vi "Wash Display Console View.vi"(8 "error in (no error)":errorcluster, 11 "View Model":T2) -> (0 "error out":errorcluster)   [LabVIEW 2017]
doc: "The Interface via which the wash controller displays the progress of the car wash.\n[Covers: UI3]"
uses:
  Model/Controls/View Model.ctl
  Model/Controls/Shared Model.ctl
  Model/Controls/Views Action.ctl
  Error Handler/Controls/Error Model.ctl
  Error Handler/Controls/Error Message.ctl
  Error Handler/Controls/Error Type.ctl
  Configuration/Controls/Config Model.ctl
  Configuration/Controls/Config DB Message.ctl
  Configuration/Controls/Config DB Command.ctl
  Configuration/Controls/Config DB Overhead.ctl
  Configuration/Controls/Config DB Record.ctl
  Controller/Controls/Controller Model.ctl
  Vehicle Position Simulation View/Controls/Vehicle - Position.ctl
  Controller/Controls/Controller Overhead.ctl
  Controller/Controls/Controller Wash Step.ctl
  Controls/Wash Display - LEDs.ctl
  Controls/Wash Display - GUI References.ctl
  Timing/Controls/Timer - Action.ctl
panel:
  out "Time Remaining":dbl format="%07.2g"
  out "Vehicle Out":bool caption="Vehicle Out of Position"
  out "Wash Entry":bool
  out "Wash LEDs":T1 caption="Car Wash Indicators"
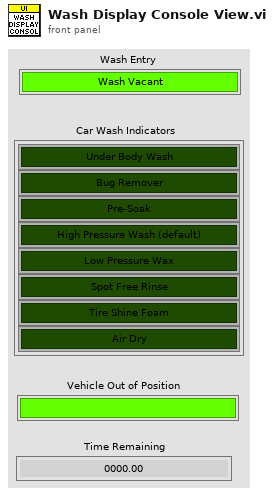
[diagram p1: front panel]
types:
  T1 = typedef "Wash Display - LEDs.ctl" = cluster{"Under Body Wash":bool, "Bug Remover":bool, "Pre-Soak":bool, "High Pressure Wash":bool, "Low Pressure Wax":bool, "Spot Free Rinse":bool, "Tire Shine Foam":bool, "Air Dry":bool}
  T2 = typedef "View Model.ctl" = cluster{"Shared Model":T3, "Error Model":T4, "Config Model":T5, "Controller Model":T6}
  T3 = typedef "Shared Model.ctl" = cluster{"Stop":refnum<user-event>, "Stop DVR":refnum<data-value>, "Views Action":refnum<user-event>}
  T4 = typedef "Error Model.ctl" = cluster{"Error":refnum<user-event>}
  T5 = typedef "Config Model.ctl" = cluster{"Config":refnum<user-event>, "Config DVR":refnum<data-value>}
  T6 = typedef "Controller Model.ctl" = cluster{"Position Change":refnum<user-event>, "Overhead DVR":refnum<data-value>, "Wash Cycle Start":refnum<user-event>, "Wash Step Start":refnum<user-event>, "Out Of Position":refnum<user-event>}
  T7 = typedef "Wash Display - GUI References.ctl" = cluster{"Time Remaining":refnum<vi>, "Vehicle Out":refnum<vi>, "Wash LEDs":refnum<vi>, "Wash Entry":refnum<vi>}
  T8 = typedef "Timer - Action.ctl" = enum16{"Start", "Get Time", "Pause", "UnPause"}
  T9 = typedef "Error Type.ctl" = enum16{"Minor Error", "Wash Cycle Error", "System Error", "Unknown"}
  T10 = typedef "Views Action.ctl" = enum16{"Initial", "Wash Cycle Start", "Wash Cycle Complete", "Wash Exit", "Wash Abort/Terminate", "Wash Step Start", "Wash Step Execute", "Wash Step Complete"}
  T11 = typedef "Controller Wash Step.ctl" = enum16{"None", "Under Body Wash", "Bug Remover", "Pre-Soak", "High Pressure Wash", "Low Pressure Wax", "Spot Free Rinse", "Tire Shine Foam", "Air Dry"}
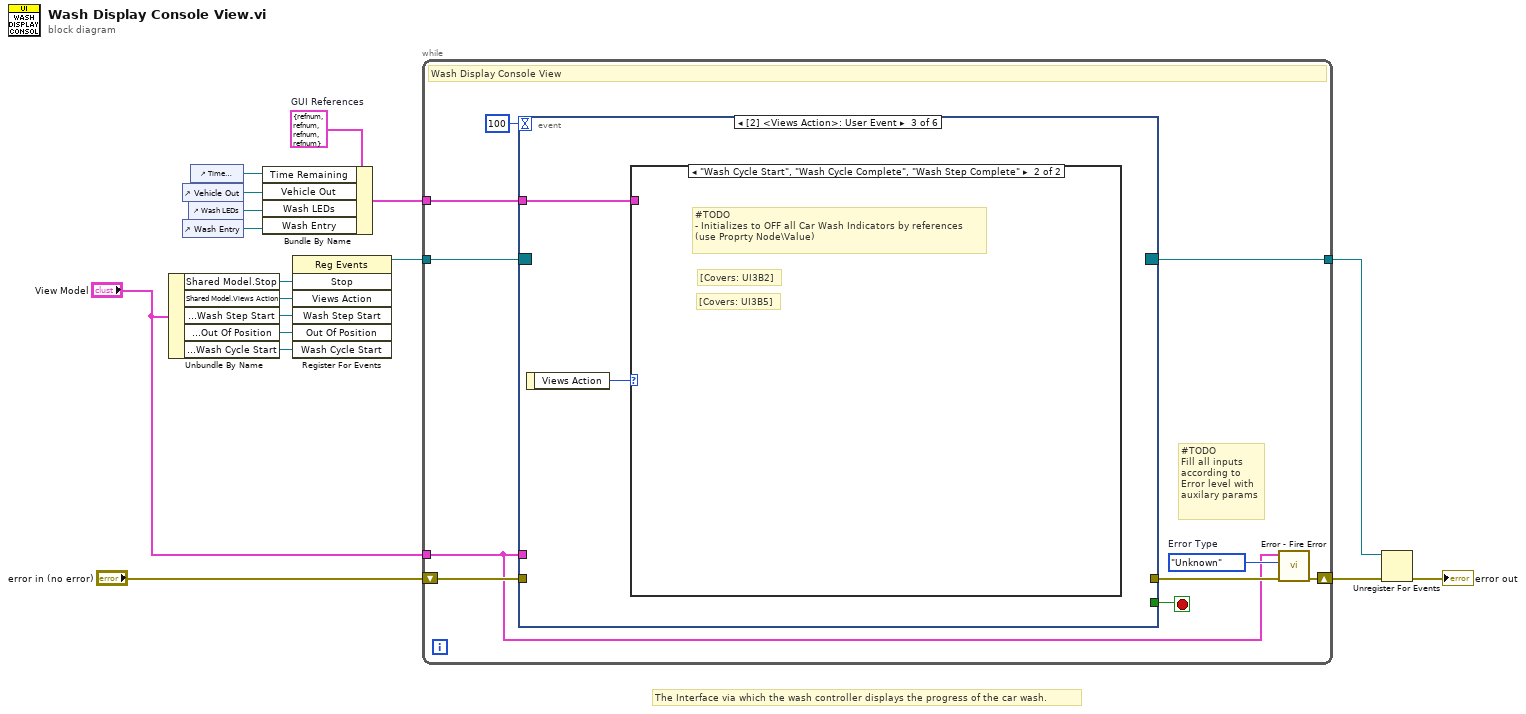
[diagram p0: block diagram]
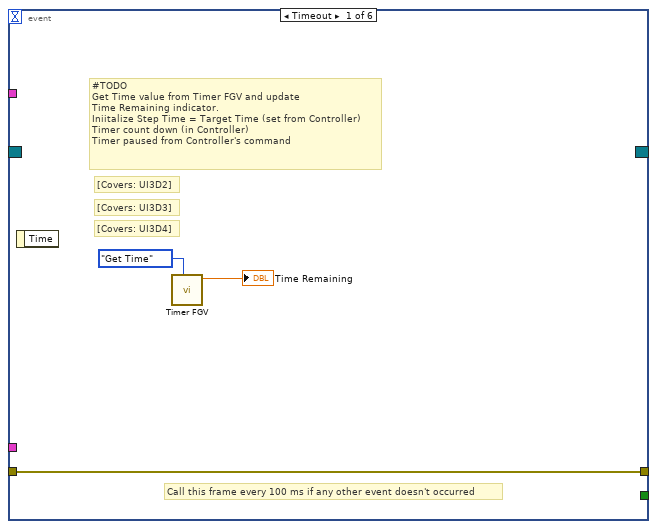
[diagram p2: hidden frame]
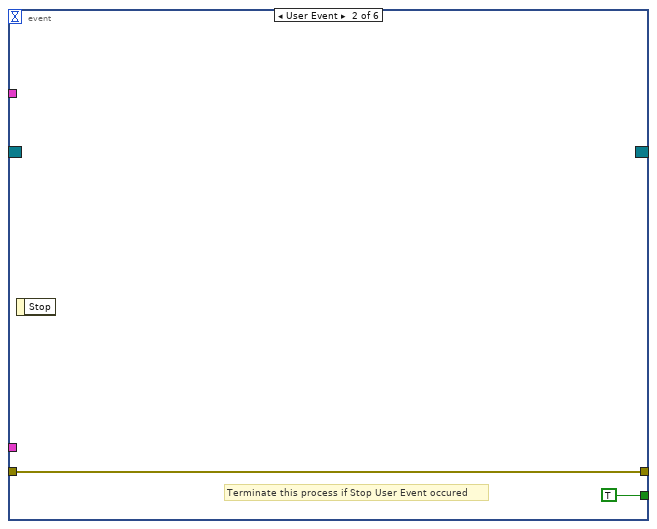
[diagram p3: hidden frame]
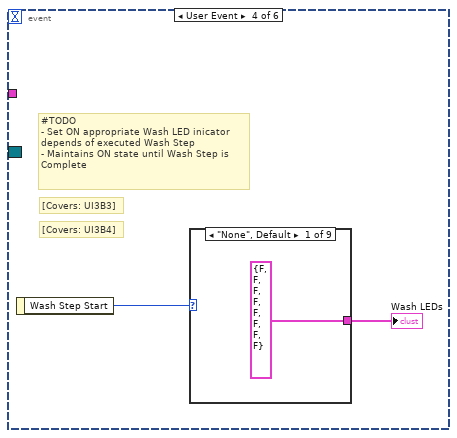
[diagram p5: hidden frame]
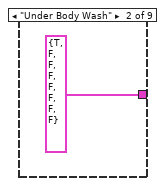
[diagram p6: hidden frame]
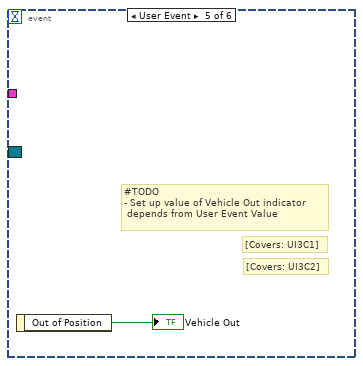
[diagram p14: hidden frame]
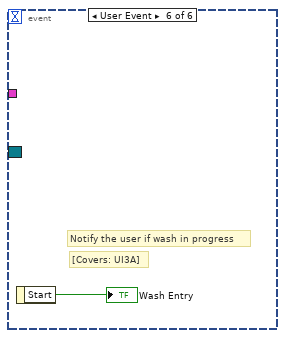
[diagram p15: hidden frame]
diagram:
  w10 = T7 {"Time Remaining"=refnum, "Vehicle Out"=refnum, "Wash LEDs"=refnum, "Wash Entry"=refnum}  # GUI References
  # "The Interface via which the wash controller displays the progress of the car wash."
  n1 = Unbundle By Name("View Model") -> ("Shared Model.Stop"=w17:refnum<user-event>, "Shared Model.Views Action"=w4:refnum<user-event>, "Controller Model.Wash Step Start"=w3:refnum<user-event>, "Controller Model.Out Of Position"=w2:refnum<user-event>, "Controller Model.Wash Cycle Start"=w1:refnum<user-event>)
  n2 = control-ref of="Vehicle Out"() -> (w8:refnum<vi>)
  n3 = control-ref of="Wash Entry"() -> (w6:refnum<vi>)
  n4 = control-ref of="Wash LEDs"() -> (w7:refnum<vi>)
  n5 = control-ref of="Time Remaining"() -> (w9:refnum<vi>)
  n6 = Bundle By Name(cluster=w10, "Time Remaining"=w9, "Vehicle Out"=w8, "Wash LEDs"=w7, "Wash Entry"=w6) -> (w5:T7)
  n7 = register-events(w17, w4, w3, w2, w1) -> (reference out=w16:refnum<event-registration>)  [unwired: 2 in, 1 out]
  n8 = while {
    tunnel: w16 -> [w27]
    shift-right: [w21] -> w14
    shift-left: "error in (no error)" -> [w25]
    tunnel: [w24] -> w12
    tunnel: "View Model" -> [w19]
    tunnel: w5 -> [w18]
    stop <- w23 stop-if-true
    w20 = Error_Type."Unknown"  # Error Type
    # "#TODO\nFill all inputs\naccording to \nError level with\nauxilary params"
    # "Wash Display Console View"
    n9 = event shown="[2] <Views Action>: User Event" {
      selector: w27 -> [_ _ _ _ _ _]
      dyn-events: [_ _ _ _ _ _] -> w24
      timeout: 100 -> [_ _ _ _ _ _]
      tunnel: w25 -> [w30 w32 _ _ _ _]
      tunnel: [w30 w32 _ _ _ _] -> w22
      tunnel: w19 -> [_ _ _ _ _ _]
      tunnel: [_ TRUE _ _ _ _] -> w23
      tunnel: w18 -> [_ _ w33 _ _ _]
      event Timeout {
        # "[Covers: UI3D4]"
        # "[Covers: UI3D3]"
        # "[Covers: UI3D2]"
        # "#TODO\nGet Time value from Timer FGV and update\nTime Remaining indicator.\nIniitalize Step Time = Target Time (set from Controller)\nTimer count down (in Controller)\nTimer paused from Controller's command"
        # "Call this frame every 100 ms if any other event doesn't occurred"
        n10 = event-data() -> ()  [unwired: 1 in, 1 out]
        n11 = call "Timer FGV.vi"("Timer Action"=Timer_-_Action."Get Time") -> ("Elapsed Time"=→"Time Remaining":dbl)  [unwired: 8 in, 2 out]
      }
      event User Event {
        # "Terminate this process if Stop User Event occured"
        n12 = event-data() -> ()  [unwired: 1 in, 1 out]
      }
      event User Event {
        n13 = event-data() -> ("Views Action"=w34:T10)  [unwired: 1 in]
        n14 = case shown="\"Wash Cycle Start\", \"Wash Cycle Complete\", \"Wash Step Complete\"" w34 {
          tunnel: w33 -> [_ _]
          frame Default {
          }
          frame "Wash Cycle Start", "Wash Cycle Complete", "Wash Step Complete" {
            # "[Covers: UI3B5]"
            # "[Covers: UI3B2]"
            # "#TODO\n- Initializes to OFF all Car Wash Indicators by references\n(use Proprty Node\\Value)"
          }
        }
      }
      event User Event {
        # "[Covers: UI3B4]"
        # "[Covers: UI3B3]"
        # "#TODO\n- Set ON appropriate Wash LED inicator\ndepends of executed Wash Step\n- Maintains ON state until Wash Step is\nComplete"
        n15 = event-data() -> ("Wash Step Start"=w36:T11)  [unwired: 1 in]
        n16 = case shown="\"None\", Default" w36 {
          tunnel: [T1 {"Under Body Wash"=FALSE, "Bug Remover"=FALSE, "Pre-Soak"=FALSE, "High Pressure Wash"=FALSE, "Low Pressure Wax"=FALSE, "Spot Free Rinse"=FALSE, "Tire Shine Foam"=FALSE, "Air Dry"=FALSE} ("Wash LEDs") T1 {"Under Body Wash"=TRUE, "Bug Remover"=FALSE, "Pre-Soak"=FALSE, "High Pressure Wash"=FALSE, "Low Pressure Wax"=FALSE, "Spot Free Rinse"=FALSE, "Tire Shine Foam"=FALSE, "Air Dry"=FALSE} ("Wash LEDs") _ _ _ _ _ _ _] -> w35
          frame "None", Default {
          }
          frame "Under Body Wash" {
          }
          frame "Bug Remover" {
          }
          frame "Pre-Soak" {
          }
          frame "High Pressure Wash" {
          }
          frame "Low Pressure Wax" {
          }
          frame "Spot Free Rinse" {
          }
          frame "Tire Shine Foam" {
          }
          frame "Air Dry" {
          }
        }
        "Wash LEDs" <- w35
      }
      event User Event {
        # "[Covers: UI3C2]"
        # "[Covers: UI3C1]"
        # "#TODO\n- Set up value of Vehicle Out indicator \n depends from User Event Value"
        n17 = event-data() -> ("Out of Position"=→"Vehicle Out":bool)  [unwired: 1 in]
      }
      event User Event {
        # "[Covers: UI3A]"
        # "Notify the user if wash in progress"
        n18 = event-data() -> ("Start"=→"Wash Entry":bool)  [unwired: 1 in]
      }
    }
    n19 = call "Error - Fire Error.vi"("error in (no error)"=w22, "Error Type"=w20, "View Model"=w19) -> ("error out"=w21:errorcluster)  [unwired: 7 in, 1 out]
  }
  n20 = Unregister For Events(event registration refnum=w12, error in=w14) -> (error out=→"error out":errorcluster)
